vi "Rinocloud_HTTP_children.vi"(3 "id":string, 5 "Tree Ref in":refnum<vi>) -> (0 "body":string, 1 "headers":string, 2 "Tree Ref out":refnum<vi>)   [LabVIEW 2013]
uses:
  Rinocloud_global_variable.vi
  <vilib>/httpClient/POSTBuffer.vi
  <vilib>/LVH/i3 JSON/JSON Parsing/Get Object Parameter Files/Get Object Parameter - Numeric.vi
  <vilib>/LVH/i3 JSON/JSON Parsing/Get Object Parameter Files/Get Object Parameter - Array.vi
  <vilib>/LVH/i3 JSON/JSON Parsing/Get Array Value at Index Files/Get Array Value at Index - Array.vi
  <vilib>/LVH/i3 JSON/JSON Parsing/Get Object Parameter Files/Get Object Parameter - String.vi
  <vilib>/httpClient/LabVIEWHTTPClient.lvlib
  i3 JSON/i3-json.lvlib
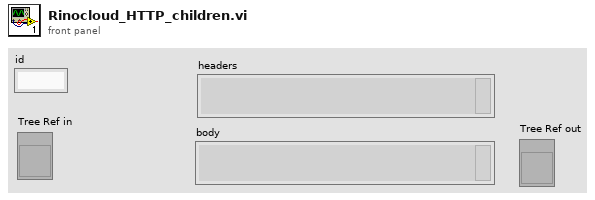
[diagram p1: front panel]
types:
  T1 = typedef "LabVIEWHTTPClient.lvlib/ClientHandle.ctl" = refnum<k1>
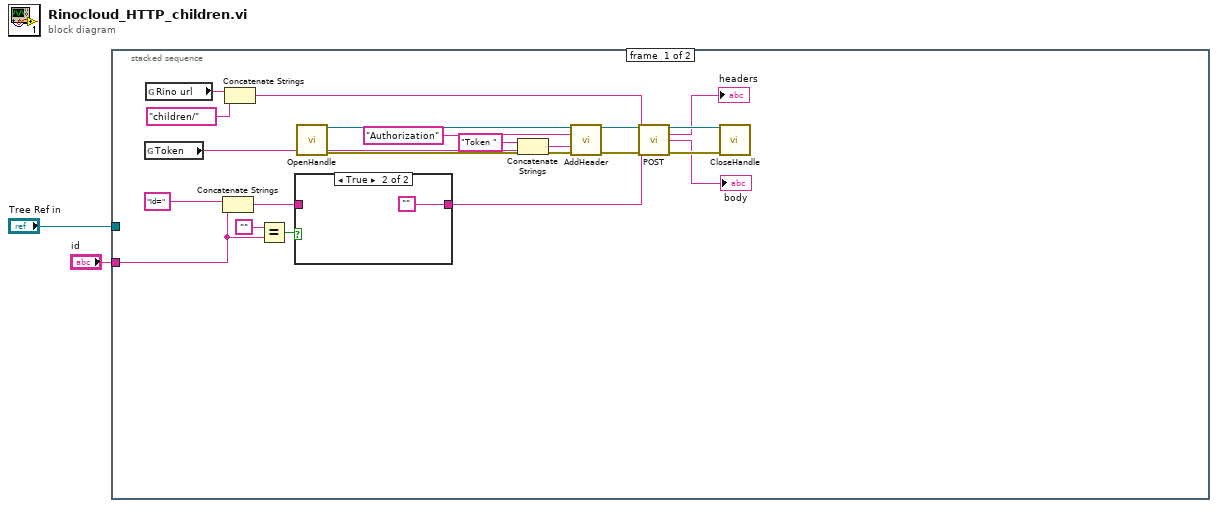
[diagram p0: block diagram]
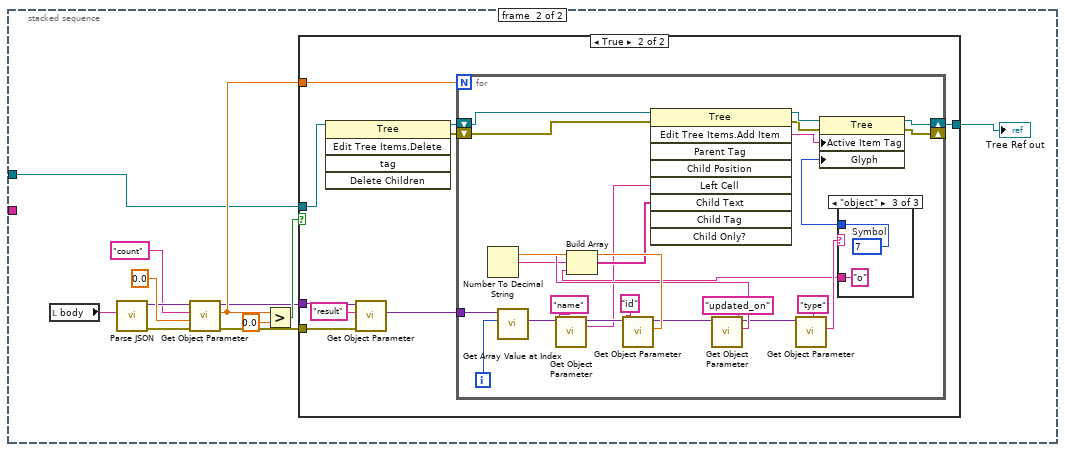
[diagram p3: hidden frame]
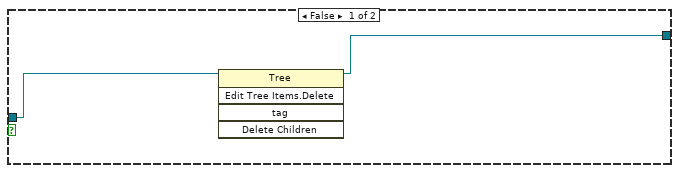
[diagram p4: hidden frame]
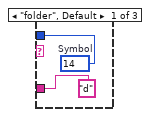
[diagram p5: hidden frame]
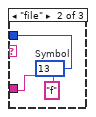
[diagram p6: hidden frame]
diagram:
  n1 = stacked-sequence {
    tunnel: "id" -> [w8 _]
    tunnel: "Tree Ref in" -> [_ w27]
    frame #0 {
      n2 = global read "Rinocloud_global_variable.vi" "Token"() -> (w15:string)
      n3 = global read "Rinocloud_global_variable.vi" "Rino url"() -> (w21:string)
      n4 = Concatenate Strings("id=" ("value"), w8) -> (w5:string)
      n5 = Concatenate Strings(w21, "children/" ("Combo Box 2")) -> (w23:string)
      n6 = Equal?(x="", y=w8) -> (x = y?=w7:bool)
      n7 = case shown="True" w7 {
        tunnel: [w24 ""] -> w6
        tunnel: w5 -> [w24 _]
        frame False {
        }
        frame True {
        }
      }
      n8 = call <vilib>:"OpenHandle.vi"() -> ("client handle out"=w19:T1, "error out"=w16:errorcluster)  [unwired: 14 in]
      n9 = Concatenate Strings("Token " ("value"), w15) -> (w17:string)
      n10 = call <vilib>:"AddHeader.vi"("client handle"=w19, "header"="Authorization" ("url"), "value"=w17, "error in (no error)"=w16) -> ("client handle out"=w12:T1, "error out"=w11:errorcluster)  [unwired: 10 in]
      n11 = call-poly <vilib>:"POST.vi"("client handle"=w12, "url"=w23, "buffer"=w6, "error in (no error)"=w11) -> ("client handle out"=w14:T1, "headers"=→"headers":string, "body"=→"body":string, "error out"=w13:errorcluster)  [unwired: 8 in]
      n12 = call <vilib>:"CloseHandle.vi"("client handle"=w14, "error in (no error)"=w13) -> ()  [unwired: 13 in, 1 out]
    }
    frame #1 {
      n13 = local read "body"() -> (w37:string)
      n14 = call <vilib>:"Parse JSON.vi"("JSON String"=w37) -> ("error out"=w29:errorcluster, "JSON Tree"=w31:variant)  [unwired: 7 in, 2 out]
      n15 = call-poly <vilib>:"Get Object Parameter.vi"("error in (no error)"=w29, "Default Value if JSON Null"=0.0, "Parameter Name"="count", "JSON Tree In (JSON Object)"=w31) -> ("error out"=w30:errorcluster, "Double Value"=w36:dbl, "JSON Tree Out Passthrough"=w32:variant)  [unwired: 4 in, 1 out]
      n16 = Greater?(x=w36, y=0.0) -> (0:w35:bool)
      n17 = case shown="True" w35 {
        tunnel: w30 -> [_ w47]
        tunnel: w32 -> [_ w46]
        tunnel: w36 -> [_ w45]
        tunnel: w27 -> [w39 w43]
        tunnel: [w38 w40] -> w26
        frame False {
          n18 = invoke class="Tree" method="Edit Tree Items.Delete"(reference=w39) -> (reference out=w38:refnum<vi>)  [unwired: 4 in, 4 out]
        }
        frame True {
          n19 = invoke class="Tree" method="Edit Tree Items.Delete"(reference=w43) -> (reference out=w42:refnum<vi>, error out=w41:errorcluster)  [unwired: 4 in, 3 out]
          n20 = call-poly <vilib>:"Get Object Parameter.vi"("error in (no error)"=w47, "Parameter Name"="result", "JSON Tree In (JSON Object)"=w46) -> ("JSON Array"=w44:variant)  [unwired: 5 in, 3 out]
          n21 = for {
            N: w45 -> [_]
            tunnel: w44 -> [w71]
            shift-right: [w53] -> w40
            shift-left: w42 -> [w59]
            shift-right: [w52] -> _
            shift-left: w41 -> [w55]
            i -> [w72]
            n22 = call-poly <vilib>:"Get Array Value at Index.vi"("Index"=w72, "JSON Tree In (JSON Array)"=w71) -> ("JSON Array"=w70:variant)  [unwired: 6 in, 3 out]
            n23 = call-poly <vilib>:"Get Object Parameter.vi"("Parameter Name"="name", "JSON Tree In (JSON Object)"=w70) -> ("String Value"=w57:string, "JSON Tree Out Passthrough"=w68:variant)  [unwired: 6 in, 2 out]
            n24 = call-poly <vilib>:"Get Object Parameter.vi"("Parameter Name"="id", "JSON Tree In (JSON Object)"=w68) -> ("Double Value"=w67:dbl, "JSON Tree Out Passthrough"=w65:variant)  [unwired: 6 in, 2 out]
            n25 = Number To Decimal String(number=w67) -> (decimal integer string=w61:string)  [unwired: 1 in]
            n26 = call-poly <vilib>:"Get Object Parameter.vi"("Parameter Name"="updated_on", "JSON Tree In (JSON Object)"=w65) -> ("String Value"=w64:string, "JSON Tree Out Passthrough"=w62:variant)  [unwired: 6 in, 2 out]
            n27 = call-poly <vilib>:"Get Object Parameter.vi"("Parameter Name"="type", "JSON Tree In (JSON Object)"=w62) -> ("String Value"=w60:string)  [unwired: 6 in, 3 out]
            n28 = case shown="\"object\"" w60 {
              tunnel: [w75 w77 w78] -> w54
              tunnel: ["d" ("Parameter Name") "f" ("Parameter Name") "o" ("Parameter Name")] -> w49
              frame "folder", Default {
                w75 = 14  # Symbol
              }
              frame "file" {
                w77 = 13  # Symbol
              }
              frame "object" {
                w78 = 7  # Symbol
              }
            }
            n29 = Build Array(w64, w61, w49) -> (w58:string[])
            n30 = invoke class="Tree" method="Edit Tree Items.Add Item"(reference=w59, error in=w55, "Left Cell"=w57, "Child Text"=w58) -> (reference out=w56:refnum<vi>, error out=w51:errorcluster, "Edit Tree Items:Add Item"=w50:string)  [unwired: 5 in, 6 out]
            n31 = property class="Tree"(reference=w56, error in=w51, "Active Item Tag"=w50, "Glyph"=w54) -> (reference out=w53:refnum<vi>, error out=w52:errorcluster)
          }
        }
      }
      "Tree Ref out" <- w26
    }
  }
